vi "Get Velocity.vi"(8 "error in (no error)":errorcluster, 11 "DC Motor Controller FPGA in":refnum<class "DC Motor Controller FPGA.lvclass">) -> (0 "error out":errorcluster, 2 "CCW Velocity (rad/s)":dbl, 3 "DC Motor Controller FPGA out":refnum<class "DC Motor Controller FPGA.lvclass">)   [LabVIEW 2013, in "DC Motor Controller FPGA.lvclass"]
doc: "Queries the counterclockwise velocity from the motor encoder."
uses:
  DC Motor Controller FPGA.lvclass
  DC Motor Controller FPGA.lvclass/DC Motor Controller FPGA.ctl
  <vilib>/rvi/interface/common/niFpgaWaitOnOcc.vi
  <vilib>/rvi/errors/niLvFpgaAdjustHostInterfaceError.vi
  <vilib>/rvi/interface/nirviReadWriteControl/nirviReadWriteControl.xnode
  NiFpgaLv.dll
  <vilib>/rvi/interface/Simulation/niFpgaSimulationCallBeginRW.vi
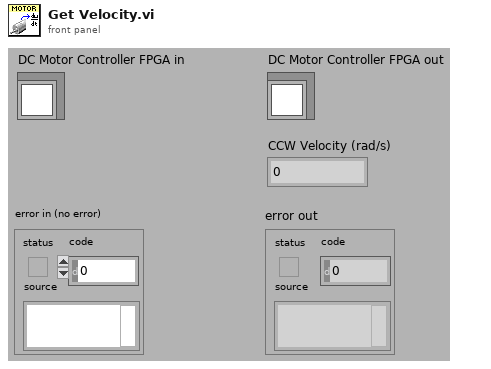
[diagram p1: front panel]
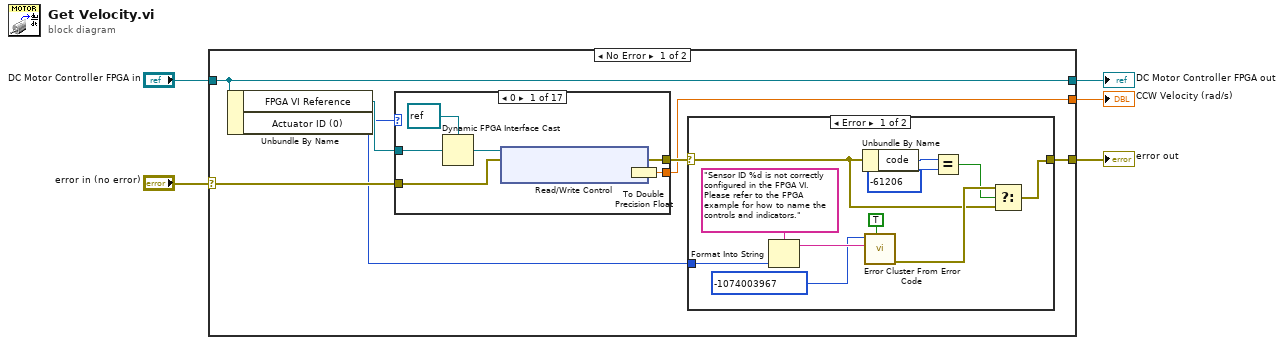
[diagram p0: block diagram]
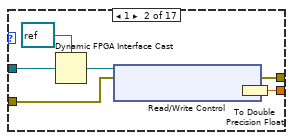
[diagram p3: hidden frame]
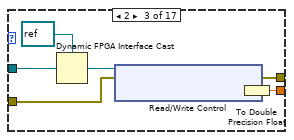
[diagram p4: hidden frame]
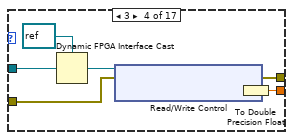
[diagram p5: hidden frame]
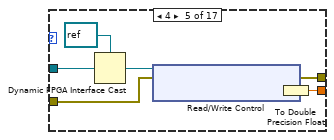
[diagram p6: hidden frame]
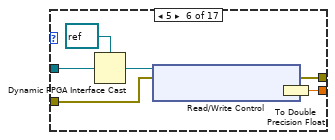
[diagram p7: hidden frame]
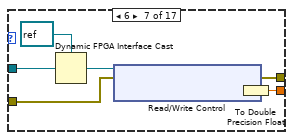
[diagram p8: hidden frame]
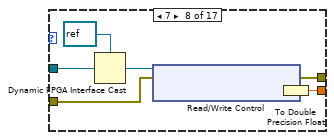
[diagram p9: hidden frame]
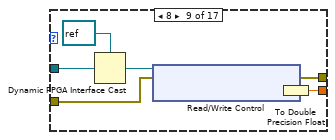
[diagram p10: hidden frame]
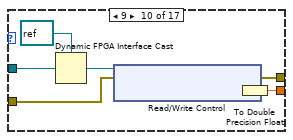
[diagram p11: hidden frame]
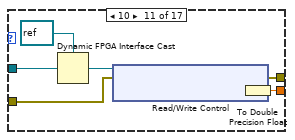
[diagram p12: hidden frame]
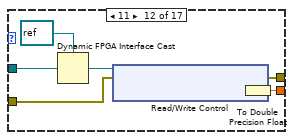
[diagram p13: hidden frame]
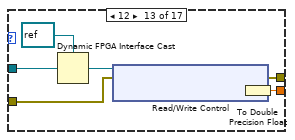
[diagram p14: hidden frame]
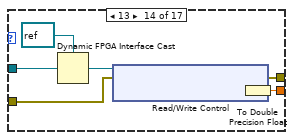
[diagram p15: hidden frame]
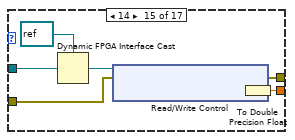
[diagram p16: hidden frame]
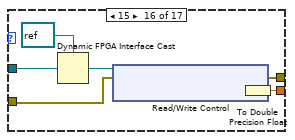
[diagram p17: hidden frame]
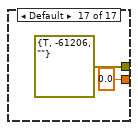
[diagram p18: hidden frame]
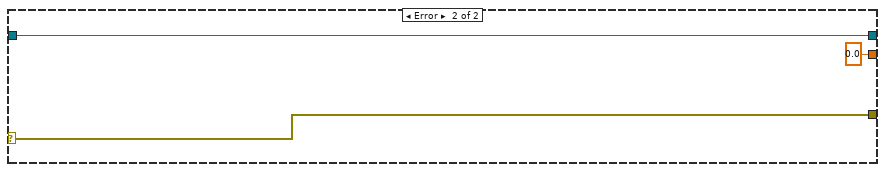
[diagram p19: hidden frame]
diagram:
  n1 = case shown="No Error" "error in (no error)" {
    selector: "error in (no error)" -> [w12 w141]
    tunnel: [w7 w141] -> w2
    tunnel: [w11 w140] -> w3
    tunnel: "DC Motor Controller FPGA in" -> [w11 w140]
    tunnel: [w6 0.0] -> w1
    frame No Error {
      n2 = Unbundle By Name(w11) -> ("FPGA VI Reference"=w10:refnum<k20>, "Actuator ID (0)"=w8:i32)
      n3 = case shown="0" w8 {
        tunnel: w10 -> [w31 w37 w44 w51 w58 w65 w72 w79 w86 w93 w100 w107 w114 w121 w128 w135 _]
        tunnel: w12 -> [w29 w36 w43 w50 w57 w64 w71 w78 w85 w91 w99 w105 w112 w119 w127 w134 _]
        tunnel: [w28 w35 w42 w49 w56 w63 w70 w77 w84 w92 w98 w106 w113 w120 w126 w133 errorcluster {"status"=TRUE, "code"=-61206, "source"=""} ("error out")] -> w9
        tunnel: [w25 w32 w40 w47 w54 w61 w68 w75 w82 w89 w95 w102 w109 w116 w124 w131 0.0] -> w6
        frame 0 {
          n4 = Dynamic FPGA Interface Cast(Session In=refnum<k20> refnum ("FPGA VI Reference Out"), Type=w31) -> (Session Out=w30:refnum<k20>)
          n5 = xnode "Read/Write Control"("FPGA VI Reference In"=w30, "error in"=w29) -> ("error out"=w28:errorcluster, "DCmotor_0_ccw vel"=w26:fxp<+/-,32,11>)  [unwired: 1 out]
          n6 = To Double Precision Float(number=w26) -> (double precision float=w25:dbl)
        }
        frame 1 {
          n7 = Dynamic FPGA Interface Cast(Session In=refnum<k20> refnum ("FPGA VI Reference Out"), Type=w37) -> (Session Out=w38:refnum<k20>)
          n8 = xnode "Read/Write Control"("FPGA VI Reference In"=w38, "error in"=w36) -> ("error out"=w35:errorcluster, "DCmotor_1_ccw vel"=w33:fxp<+/-,32,11>)  [unwired: 1 out]
          n9 = To Double Precision Float(number=w33) -> (double precision float=w32:dbl)
        }
        frame 2 {
          n10 = Dynamic FPGA Interface Cast(Session In=refnum<k20> refnum ("FPGA VI Reference Out"), Type=w44) -> (Session Out=w45:refnum<k20>)
          n11 = xnode "Read/Write Control"("FPGA VI Reference In"=w45, "error in"=w43) -> ("error out"=w42:errorcluster, "DCmotor_2_ccw vel"=w39:fxp<+/-,32,11>)  [unwired: 1 out]
          n12 = To Double Precision Float(number=w39) -> (double precision float=w40:dbl)
        }
        frame 3 {
          n13 = Dynamic FPGA Interface Cast(Session In=refnum<k20> refnum ("FPGA VI Reference Out"), Type=w51) -> (Session Out=w52:refnum<k20>)
          n14 = xnode "Read/Write Control"("FPGA VI Reference In"=w52, "error in"=w50) -> ("error out"=w49:errorcluster, "DCmotor_3_ccw vel"=w46:fxp<+/-,32,11>)  [unwired: 1 out]
          n15 = To Double Precision Float(number=w46) -> (double precision float=w47:dbl)
        }
        frame 4 {
          n16 = Dynamic FPGA Interface Cast(Session In=refnum<k20> refnum ("FPGA VI Reference Out"), Type=w58) -> (Session Out=w59:refnum<k20>)
          n17 = xnode "Read/Write Control"("FPGA VI Reference In"=w59, "error in"=w57) -> ("error out"=w56:errorcluster, "DCmotor_4_ccw vel"=w53:fxp<+/-,32,11>)  [unwired: 1 out]
          n18 = To Double Precision Float(number=w53) -> (double precision float=w54:dbl)
        }
        frame 5 {
          n19 = Dynamic FPGA Interface Cast(Session In=refnum<k20> refnum ("FPGA VI Reference Out"), Type=w65) -> (Session Out=w66:refnum<k20>)
          n20 = xnode "Read/Write Control"("FPGA VI Reference In"=w66, "error in"=w64) -> ("error out"=w63:errorcluster, "DCmotor_5_ccw vel"=w60:fxp<+/-,32,11>)  [unwired: 1 out]
          n21 = To Double Precision Float(number=w60) -> (double precision float=w61:dbl)
        }
        frame 6 {
          n22 = Dynamic FPGA Interface Cast(Session In=refnum<k20> refnum ("FPGA VI Reference Out"), Type=w72) -> (Session Out=w73:refnum<k20>)
          n23 = xnode "Read/Write Control"("FPGA VI Reference In"=w73, "error in"=w71) -> ("error out"=w70:errorcluster, "DCmotor_6_ccw vel"=w67:fxp<+/-,32,11>)  [unwired: 1 out]
          n24 = To Double Precision Float(number=w67) -> (double precision float=w68:dbl)
        }
        frame 7 {
          n25 = Dynamic FPGA Interface Cast(Session In=refnum<k20> refnum ("FPGA VI Reference Out"), Type=w79) -> (Session Out=w80:refnum<k20>)
          n26 = xnode "Read/Write Control"("FPGA VI Reference In"=w80, "error in"=w78) -> ("error out"=w77:errorcluster, "DCmotor_7_ccw vel"=w74:fxp<+/-,32,11>)  [unwired: 1 out]
          n27 = To Double Precision Float(number=w74) -> (double precision float=w75:dbl)
        }
        frame 8 {
          n28 = Dynamic FPGA Interface Cast(Session In=refnum<k20> refnum ("FPGA VI Reference Out"), Type=w86) -> (Session Out=w87:refnum<k20>)
          n29 = xnode "Read/Write Control"("FPGA VI Reference In"=w87, "error in"=w85) -> ("error out"=w84:errorcluster, "DCmotor_8_ccw vel"=w81:fxp<+/-,32,11>)  [unwired: 1 out]
          n30 = To Double Precision Float(number=w81) -> (double precision float=w82:dbl)
        }
        frame 9 {
          n31 = Dynamic FPGA Interface Cast(Session In=refnum<k20> refnum ("FPGA VI Reference Out"), Type=w93) -> (Session Out=w94:refnum<k20>)
          n32 = xnode "Read/Write Control"("FPGA VI Reference In"=w94, "error in"=w91) -> ("error out"=w92:errorcluster, "DCmotor_9_ccw vel"=w88:fxp<+/-,32,11>)  [unwired: 1 out]
          n33 = To Double Precision Float(number=w88) -> (double precision float=w89:dbl)
        }
        frame 10 {
          n34 = Dynamic FPGA Interface Cast(Session In=refnum<k20> refnum ("FPGA VI Reference Out"), Type=w100) -> (Session Out=w101:refnum<k20>)
          n35 = xnode "Read/Write Control"("FPGA VI Reference In"=w101, "error in"=w99) -> ("error out"=w98:errorcluster, "DCmotor_10_ccw vel"=w96:fxp<+/-,32,11>)  [unwired: 1 out]
          n36 = To Double Precision Float(number=w96) -> (double precision float=w95:dbl)
        }
        frame 11 {
          n37 = Dynamic FPGA Interface Cast(Session In=refnum<k20> refnum ("FPGA VI Reference Out"), Type=w107) -> (Session Out=w108:refnum<k20>)
          n38 = xnode "Read/Write Control"("FPGA VI Reference In"=w108, "error in"=w105) -> ("error out"=w106:errorcluster, "DCmotor_11_ccw vel"=w103:fxp<+/-,32,11>)  [unwired: 1 out]
          n39 = To Double Precision Float(number=w103) -> (double precision float=w102:dbl)
        }
        frame 12 {
          n40 = Dynamic FPGA Interface Cast(Session In=refnum<k20> refnum ("FPGA VI Reference Out"), Type=w114) -> (Session Out=w115:refnum<k20>)
          n41 = xnode "Read/Write Control"("FPGA VI Reference In"=w115, "error in"=w112) -> ("error out"=w113:errorcluster, "DCmotor_12_ccw vel"=w110:fxp<+/-,32,11>)  [unwired: 1 out]
          n42 = To Double Precision Float(number=w110) -> (double precision float=w109:dbl)
        }
        frame 13 {
          n43 = Dynamic FPGA Interface Cast(Session In=refnum<k20> refnum ("FPGA VI Reference Out"), Type=w121) -> (Session Out=w122:refnum<k20>)
          n44 = xnode "Read/Write Control"("FPGA VI Reference In"=w122, "error in"=w119) -> ("error out"=w120:errorcluster, "DCmotor_13_ccw vel"=w117:fxp<+/-,32,11>)  [unwired: 1 out]
          n45 = To Double Precision Float(number=w117) -> (double precision float=w116:dbl)
        }
        frame 14 {
          n46 = Dynamic FPGA Interface Cast(Session In=refnum<k20> refnum ("FPGA VI Reference Out"), Type=w128) -> (Session Out=w129:refnum<k20>)
          n47 = xnode "Read/Write Control"("FPGA VI Reference In"=w129, "error in"=w127) -> ("error out"=w126:errorcluster, "DCmotor_14_ccw vel"=w123:fxp<+/-,32,11>)  [unwired: 1 out]
          n48 = To Double Precision Float(number=w123) -> (double precision float=w124:dbl)
        }
        frame 15 {
          n49 = Dynamic FPGA Interface Cast(Session In=refnum<k20> refnum ("FPGA VI Reference Out"), Type=w135) -> (Session Out=w136:refnum<k20>)
          n50 = xnode "Read/Write Control"("FPGA VI Reference In"=w136, "error in"=w134) -> ("error out"=w133:errorcluster, "DCmotor_15_ccw vel"=w130:fxp<+/-,32,11>)  [unwired: 1 out]
          n51 = To Double Precision Float(number=w130) -> (double precision float=w131:dbl)
        }
        frame Default {
        }
      }
      n52 = case shown="Error" w9 {
        selector: w9 -> [w13 w24]
        tunnel: w8 -> [w16 _]
        tunnel: [w15 w24] -> w7
        frame Error {
          n53 = Format Into String(format string="Sensor ID %d is not correctly configured in the FPGA VI. Please refer to the FPGA example for how to name the controls and indicators." ("Source (VI Name)"), w16) -> (resulting string=w20:string)  [unwired: 2 in, 1 out]
          n54 = Unbundle By Name(w13) -> ("code"=w21:i32)
          n55 = call <vilib>:"Error Cluster From Error Code.vi"("show call chain? (False)"=TRUE, "error message (\"\")"=w20, "error code (0)"=-1074003967 ("Code")) -> ("error out"=w23:errorcluster)  [unwired: 6 in]
          n56 = Equal?(x=w21, y=-61206) -> (x = y?=w22:bool)
          n57 = Select(t=w23, s=w22, f=w13) -> (s? t:f=w15:errorcluster)
        }
        frame No Error {
        }
      }
    }
    frame Error {
    }
  }
  "error out" <- w2
  "DC Motor Controller FPGA out" <- w3
  "CCW Velocity (rad/s)" <- w1
